vi "get_status_warmedup.vi"(8 "error in (no error)":errorcluster, 11 "LightSourceMH110124MaiTai in":refnum<class "LightSourceMH110124MaiTai.lvclass">) -> (0 "error out":errorcluster, 1 "percentage warm":dbl, 2 "warmed up?":bool, 3 "LightSourceMH110124MaiTai out":refnum<class "LightSourceMH110124MaiTai.lvclass">)   [LabVIEW 2010, in "LightSourceMH110124MaiTai.lvclass"]
uses:
  LightSourceMH110124MaiTai.lvclass
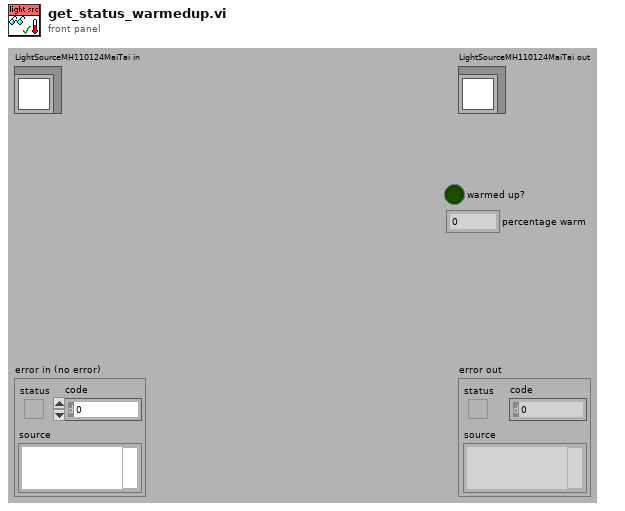
[diagram p1: front panel]
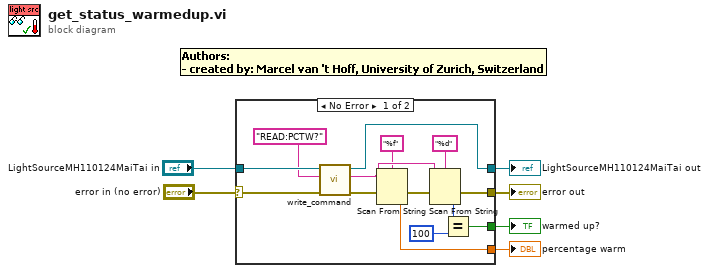
[diagram p0: block diagram]
diagram:
  n1 = case shown="No Error" "error in (no error)" {
    selector: "error in (no error)" -> [w19 w22]
    tunnel: [w18 w22] -> w2
    tunnel: [w17 w21] -> w5
    tunnel: "LightSourceMH110124MaiTai in" -> [w20 w21]
    tunnel: [w12 _] -> w4
    tunnel: [w7 _] -> w3
    frame No Error {
      n2 = call-dynamic "write_command.vi"("error in (no error)"=w19, "string to write"="READ:PCTW?", "LightSourceMH110124MaiTai in"=w20) -> ("error out"=w11:errorcluster, "read string"=w9:string, "LightSourceMH110124MaiTai out"=w17:refnum<class "LightSourceMH110124MaiTai.lvclass">)  [unwired: 6 in]
      n3 = Scan From String(format string="%f", input string=w9, error in=w11) -> (error out=w10:errorcluster, output 1=w7:dbl)  [unwired: 2 in, 2 out]
      n4 = Scan From String(format string="%d", input string=w9, error in=w10) -> (error out=w18:errorcluster, output 1=w13:i32)  [unwired: 2 in, 2 out]
      n5 = Equal?(x=w13, y=100) -> (x = y?=w12:bool)
    }
    frame Error {
    }
  }
  "error out" <- w2
  "LightSourceMH110124MaiTai out" <- w5
  "percentage warm" <- w3
  "warmed up?" <- w4
